vi "p2.vi"() -> ()   [LabVIEW 2021, in "d16.lvlib"]
uses:
  d16.lvlib
  Volcano/Volcano.lvclass
  Volcano/Volcano.lvclass/Volcano.ctl
  AOC/AOC.lvlib
panel:
  out "Solution Number":i32
  out "Number of Solutions":i32
  out "Waveform Chart 2":i32(graph)
  out "Waveform Chart":i32(graph)
  out "max value":u64
  out "# elements in elephant's queue":i32
  out "elephant's Iterations":i32=40293
  out "# elements in my queue":i32
  out "my iterations":i32=40293
  in  "Max Time":i32=26
  in  "Example":string="Valve AA has flow rate=0; tunnels lead to valves DD, II, BB\nValve BB has flow rate=13; tunnels lead to valves CC, AA\nValve CC has flow rate=2; tunnels lead to valves DD, BB\nValve DD has flow rate=20; tunnels lead to valves CC, AA, EE\nValve EE has flow rate=3; tunnels lead to valves FF, DD\nValve FF has flow rate=0; tunnels lead to valves EE, GG\nValve GG has flow rate=0; tunnels lead to valves FF, HH\nValve HH has flow rate=22; tunnel leads to valve GG\nValve II has flow rate=0; tunnels lead to valves AA, JJ\nValve JJ has flow rate=21; tunnel leads to valve II"
  in  "Example":bool=TRUE
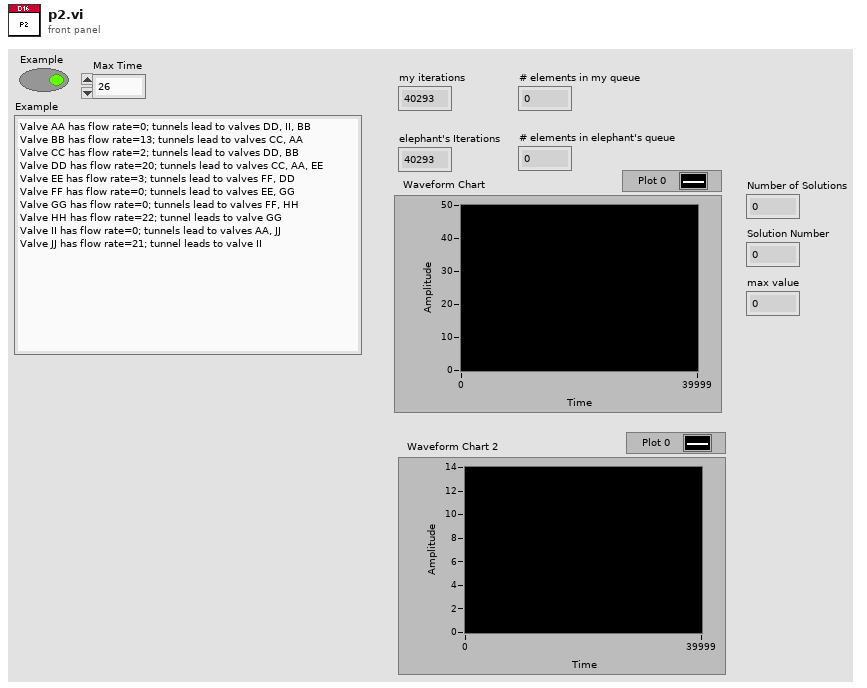
[diagram p1: front panel]
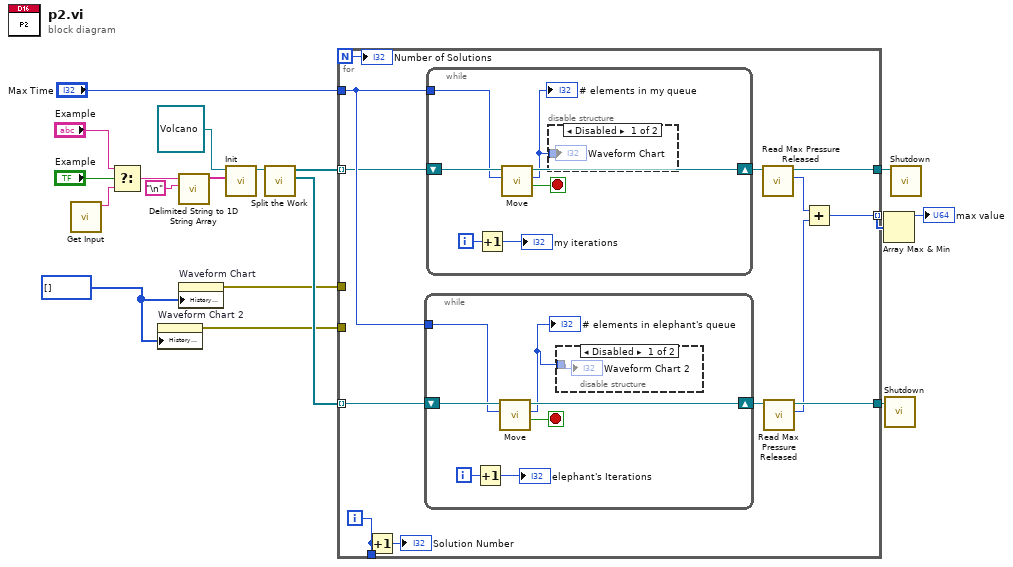
[diagram p0: block diagram]
diagram:
  w3 = i32[] [] ("History Data")
  n1 = call "Get Input.vi"() -> ("Input"=w18:string)  [unwired: 11 in]
  n2 = Select(t="Example", s="Example", f=w18) -> (s? t:f=w17:string)
  n3 = property on="Waveform Chart 2" class="WFChart (strict)"("History Data"=w3) -> (error out=w1:errorcluster)  [unwired: 2 in, 1 out]
  n4 = call <vilib>:"Delimited String to 1D String Array.vi"("delimiter"="\n", "delimited string"=w17) -> ("string array"=w12:string[])  [unwired: 9 in]
  n5 = property on="Waveform Chart" class="WFChart (strict)"("History Data"=w3) -> (error out=w2:errorcluster)  [unwired: 2 in, 1 out]
  n6 = call "Init.vi"("input"=w12, "Volcano in"=refnum<class "Volcano.lvclass"> refnum ("d16.lvlib:Volcano.lvclass")) -> ("Volcano out"=w10:refnum<class "Volcano.lvclass">)  [unwired: 9 in]
  n7 = call "Split the Work.vi"("Volcano"=w10) -> ("Elephant's Volcanoes"=w8:refnum<class "Volcano.lvclass">[], "My Volcanoes"=w9:refnum<class "Volcano.lvclass">[])  [unwired: 9 in]
  n8 = for {
    N -> [w20]
    tunnel: "Max Time" -> [w30]
    tunnel: w9 -> [w29] mode=indexing
    tunnel: w8 -> [w28] mode=indexing
    tunnel: [w23] -> w5 mode=indexing
    tunnel: [w26] -> w7
    tunnel: [w25] -> w6
    tunnel: [w24] -> _
    tunnel: w2 -> [_]
    tunnel: w1 -> [_]
    i -> [w24]
    n9 = Increment(x=w24) -> (x+1=→"Solution Number":i32)
    n10 = while {
      shift-right: [w37] -> w21
      shift-left: w28 -> [w38]
      tunnel: w30 -> [w36]
      i -> [w34]
      stop <- w35 stop-if-true
      n11 = Increment(x=w34) -> (x+1=→"elephant's Iterations":i32)
      n12 = call "Move.vi"("max time"=w36, "Volcano in"=w38) -> ("Finished?"=w35:bool, "# elements in queue"=w32:i32, "Volcano out"=w37:refnum<class "Volcano.lvclass">)  [unwired: 7 in]
      "# elements in elephant's queue" <- w32
      n13 = disable-structure shown="Disabled" {
        disable-tunnel: w32 -> [w39 _]
        frame Disabled {
          "Waveform Chart 2" <- w39
        }
        frame Enabled {
        }
      }
    }
    n14 = while {
      shift-right: [w45] -> w31
      shift-left: w29 -> [w46]
      tunnel: w30 -> [w44]
      i -> [w42]
      stop <- w43 stop-if-true
      n15 = Increment(x=w42) -> (x+1=→"my iterations":i32)
      n16 = call "Move.vi"("max time"=w44, "Volcano in"=w46) -> ("Finished?"=w43:bool, "# elements in queue"=w40:i32, "Volcano out"=w45:refnum<class "Volcano.lvclass">)  [unwired: 7 in]
      "# elements in my queue" <- w40
      n17 = disable-structure shown="Disabled" {
        disable-tunnel: w40 -> [w47 _]
        frame Disabled {
          "Waveform Chart" <- w47
        }
        frame Enabled {
        }
      }
    }
    n18 = call "Read Max Pressure Released.vi"("Volcano in"=w31) -> ("Max Pressure Released"=w27:u64, "Volcano out"=w26:refnum<class "Volcano.lvclass">)  [unwired: 9 in]
    n19 = call "Read Max Pressure Released.vi"("Volcano in"=w21) -> ("Max Pressure Released"=w22:u64, "Volcano out"=w25:refnum<class "Volcano.lvclass">)  [unwired: 9 in]
    n20 = Add(x=w27, y=w22) -> (x+y=w23:u64)
    "Number of Solutions" <- w20
  }
  n21 = Array Max & Min(array=w5) -> (max value=→"max value":u64)  [unwired: 3 out]
  n22 = call "Shutdown.vi"("Volcano in"=w6) -> ()  [unwired: 10 in, 1 out]
  n23 = call "Shutdown.vi"("Volcano in"=w7) -> ()  [unwired: 10 in, 1 out]
